vi "Calculate Linear Sweep.vi"(9 "Points":i32, 10 "Stop level":dbl, 11 "Start level":dbl) -> (3 "Values":dbl[](array[numeric]))   [LabVIEW 2021, in "PMIC Common.lvlib"]
uses:
  PMIC Common.lvlib
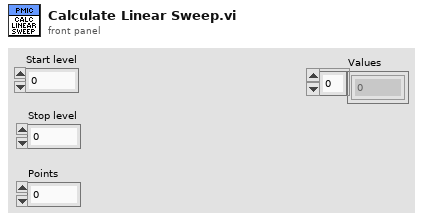
[diagram p1: front panel]
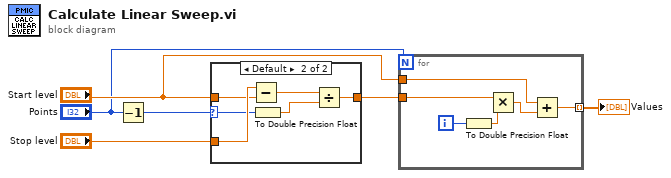
[diagram p0: block diagram]
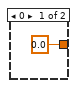
[diagram p2: hidden frame]
diagram:
  n1 = Decrement(x="Points") -> (x-1=w3:i32)
  n2 = case shown="Default" w3 {
    selector: w3 -> [_ w8]
    tunnel: "Stop level" -> [_ w13]
    tunnel: "Start level" -> [_ w12]
    tunnel: [0.0 w10] -> w2
    frame 0 {
    }
    frame Default {
      n3 = Subtract(x=w13, y=w12) -> (x-y=w11:dbl)
      n4 = To Double Precision Float(number=w8) -> (double precision float=w9:dbl)
      n5 = Divide(x=w11, y=w9) -> (x/y=w10:dbl)
    }
  }
  n6 = for {
    N: "Points" -> [_]
    tunnel: w2 -> [w19]
    tunnel: "Start level" -> [w14]
    tunnel: [w16] -> w1 mode=indexing
    i -> [w18]
    n7 = To Double Precision Float(number=w18) -> (double precision float=w17:dbl)
    n8 = Multiply(x=w19, y=w17) -> (x*y=w15:dbl)
    n9 = Add(x=w14, y=w15) -> (x+y=w16:dbl)
  }
  "Values" <- w1
